vi "onExportResults.vi"(8 "error in (no error)":errorcluster, 11 "Pips in":refnum<class "Pips.lvclass">) -> (0 "error out":errorcluster, 3 "Pips out":refnum<class "Pips.lvclass">)   [LabVIEW 2021, in "Bananas.lvlib" / "Pips.lvclass"]
uses:
  Pips.lvclass
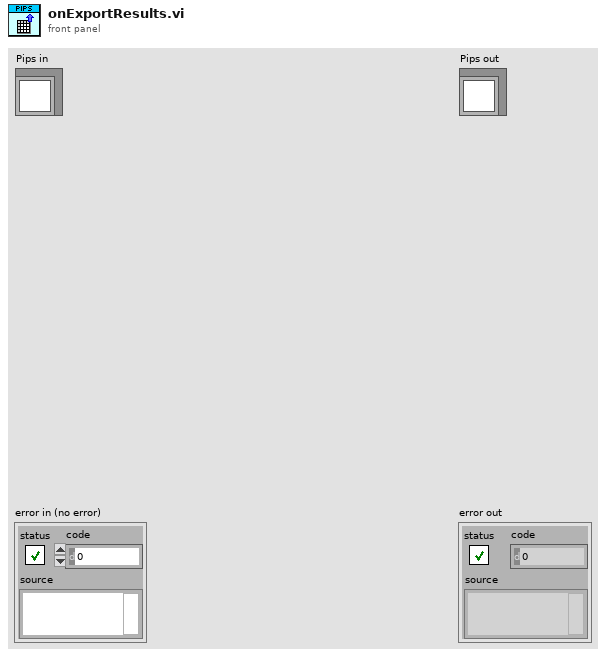
[diagram p1: front panel]
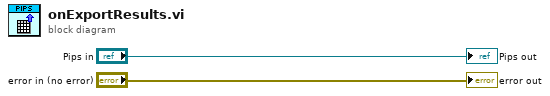
[diagram p0: block diagram]
diagram:
  "error out" <- "error in (no error)"
  "Pips out" <- "Pips in"
